vi "Append.vi"(8 "error in (no error)":errorcluster, 9 "Runnable":refnum<class "Runnable.lvclass">, 10 "Name":string, 11 "LUnit Test Suite In":refnum<class "LUnit Test Suite.lvclass">) -> (0 "error out":errorcluster, 3 "LUnit Test Suite Out":refnum<class "LUnit Test Suite.lvclass">)   [LabVIEW 2020, in "LUnit Test Suite.lvclass"]
uses:
  LUnit Test Suite.lvclass
  Runnable/Runnable.lvclass
  LUnit Test Suite.lvclass/LUnit Test Suite.ctl
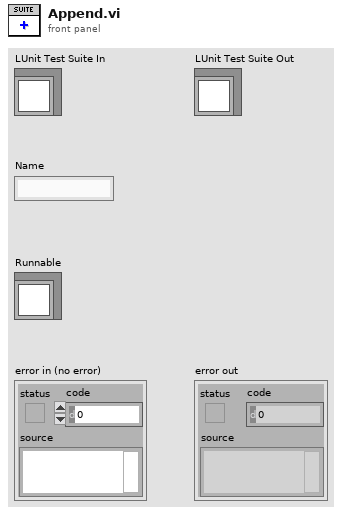
[diagram p1: front panel]
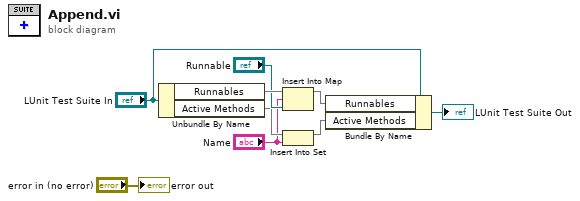
[diagram p0: block diagram]
diagram:
  n1 = Unbundle By Name("LUnit Test Suite In") -> ("Runnables"=w6:map{string, refnum<class "Runnable.lvclass">}, "Active Methods"=w2:set{string})
  n2 = Insert Into Map(map in=w6, key="Name", value="Runnable") -> (map out=w5:map{string, refnum<class "Runnable.lvclass">})  [unwired: 2 out]
  n3 = Insert Into Set(10:"Name", 11:w2) -> (3:w3:set{string})  [unwired: 1 out]
  n4 = Bundle By Name(cluster="LUnit Test Suite In", "Runnables"=w5, "Active Methods"=w3) -> (→"LUnit Test Suite Out":refnum<class "LUnit Test Suite.lvclass">)
  "error out" <- "error in (no error)"
